vi "MindwaveGetPAYLOAD.vi"(4 "error input":errorcluster, 6 "[PLENGTH]":u8, 7 "VISA resource name input":refnum<visa-resource-name>) -> (0 "error out":errorcluster, 1 "[PAYLOAD]":u8[](array[numeric]) format="%x", 2 "[CHECKSUM]":u8 format="%x", 3 "VISA resource name out":refnum<visa-resource-name>)   [LabVIEW 2011, in "Neurosky.lvlib"]
uses:
  Users/Isaias/Documents/GitHub/Neurosky/Neurosky.lvlib
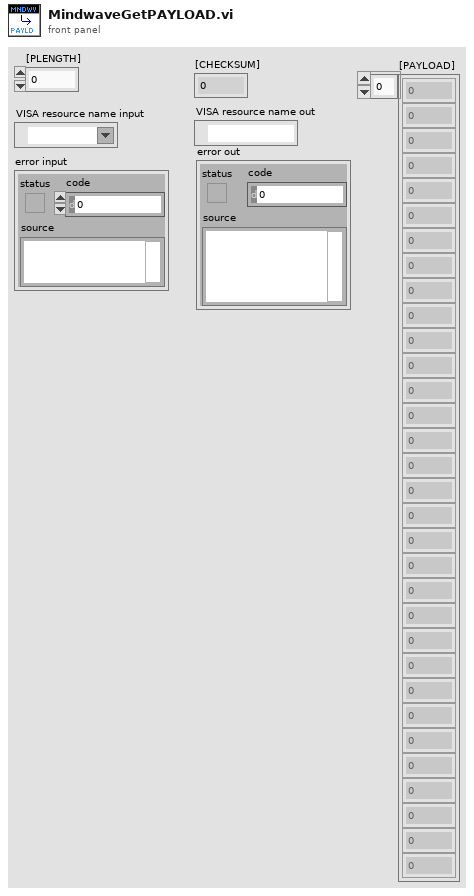
[diagram p1: front panel]
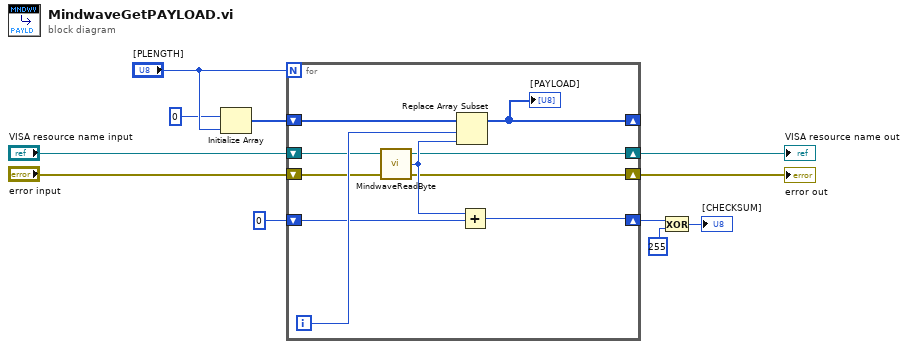
[diagram p0: block diagram]
diagram:
  n1 = Initialize Array(u8 0 ("element"), "[PLENGTH]") -> (w3:u8[])
  n2 = for {
    N: "[PLENGTH]" -> [_]
    shift-right: [w17] -> _
    shift-left: w3 -> [w20]
    shift-right: [w19] -> w5
    shift-left: u16 0 ("element") -> [w18]
    shift-right: [w15] -> w10
    shift-left: "error input" -> [w12]
    shift-right: [w14] -> w11
    shift-left: "VISA resource name input" -> [w13]
    i -> [w21]
    n3 = call <userlib>:"MindwaveReadByte.vi"("error in (no error) input"=w12, "VISA resource name input"=w13) -> ("error out"=w15:errorcluster, "byte"=w16:u8, "VISA resource name out"=w14:refnum<visa-resource-name>)  [unwired: 2 in]
    n4 = Replace Array Subset(array=w20, new element=w16, index=w21) -> (w17:u8[])
    "[PAYLOAD]" <- w17
    n5 = Add(x=w16, y=w18) -> (x+y=w19:u16)
  }
  "VISA resource name out" <- w11
  "error out" <- w10
  n6 = Exclusive Or(1:u8 255 ("element"), 2:w5) -> (0:→"[CHECKSUM]":u16)
